vi "TCP Flush.vi"(8 "Error In":errorcluster, 11 "LINX Device Config":T1={"Interface"=enum."TCP", "COM Port"="COM5", "TCP Configuration"={"IP Address"="10.2.106.213", "Port"=6921}, "Device Family"=enum."Digilent", "Device ID"=1, "Device Name"="chipKIT uC32", "TCP Ref"=refnum}) -> (0 "Error Out":errorcluster, 2 "Flushed Data":string, 3 "LINX Device Config":T1={"Interface"=enum."TCP", "COM Port"="COM5", "TCP Configuration"={"IP Address"="10.2.106.213", "Port"=6921}, "Device Family"=enum."Digilent", "Device ID"=1, "Device Name"="chipKIT uC32", "TCP Ref"=refnum})   [LabVIEW 2013, in "LVH-LINX.lvlib" / "Device.lvlib"]
uses:
  <vilib>/LabVIEW Hacker/LINX/Private/Device/Device.lvlib
  <vilib>/LabVIEW Hacker/LINX/Private/Device/Type Defs/LINX Device Config.ctl
  <vilib>/LabVIEW Hacker/LINX/Private/Type Defs/Interface.ctl
  <vilib>/LabVIEW Hacker/LINX/Private/Device/Type Defs/TCP Config.ctl
  <vilib>/LabVIEW Hacker/LINX/Private/Type Defs/Device Family.ctl
  <vilib>/LabVIEW Hacker/LINX/LVH-LINX.lvlib
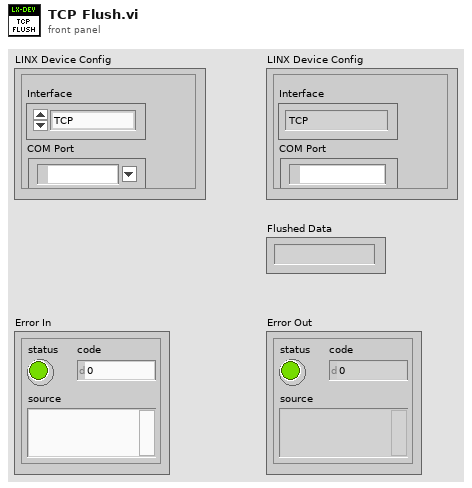
[diagram p1: front panel]
types:
  T1 = typedef "LVH-LINX.lvlib/Device.lvlib/LINX Device Config.ctl" = cluster{"Interface":T2, "COM Port":refnum<visa-resource-name>, "TCP Configuration":T3, "Device Family":T4, "Device ID":u8, "Device Name":string, "TCP Ref":refnum<k5>}
  T2 = typedef "LVH-LINX.lvlib/Interface.ctl" = enum16{"Serial", "TCP"}
  T3 = typedef "LVH-LINX.lvlib/Device.lvlib/TCP Config.ctl" = cluster{"IP Address":string, "Port":u16}
  T4 = typedef "LVH-LINX.lvlib/Device Family.ctl" = enum8{"National Instruments", "Digilent", "Arduino"}
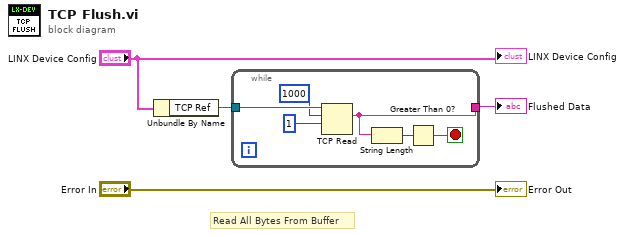
[diagram p0: block diagram]
diagram:
  # "Read All Bytes From Buffer"
  n1 = Unbundle By Name("LINX Device Config") -> ("TCP Ref"=w4:refnum<k5>)
  n2 = while {
    tunnel: w4 -> [w10]
    tunnel: [w5] -> w1
    stop <- w6 stop-if-true
    n3 = TCP Read(connection ID=w10, bytes to read=1000, 9:1 ("timeout ms (25000)")) -> (data out=w5:string)  [unwired: 2 in, 2 out]
    n4 = String Length(string=w5) -> (length=w7:i32)
    n5 = Greater Than 0?(x=w7) -> (x > 0?=w6:bool)
  }
  "Flushed Data" <- w1
  "Error Out" <- "Error In"
  "LINX Device Config" <- "LINX Device Config"
